vi "QueryNTPparse.vi"(0 "IP Address of NIST Server":string="132.163.4.102", 1 "error in (no error)":errorcluster) -> (2 "NTP Time":u64, 3 "time stamp UTC":timestamp, 4 "error out":errorcluster)   [LabVIEW 2012]
panel:
  out "time stamp NTP":timestamp
  out "time stamp":timestamp
  out "raw data":string
  # "This is a first draft to query an NTP server (proof of concept).\nhttp://forums.ni.com/ni/board/message?board.id=170&message.id=458949&jump=true"
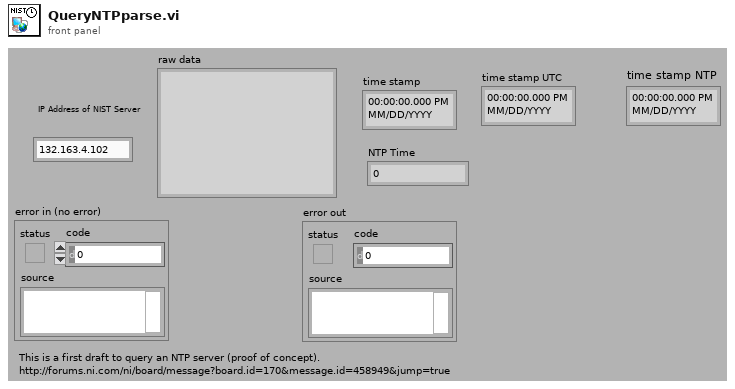
[diagram p1: front panel]
types:
  T1 = cluster{"LI|VM|Mode":u8, "Stratum":u8, "Poll":u8, "Precision":u8, "Root Delay":u32, "Root Dispersion":u32, "Reference Identifier":u32, "Reference Timestamp":fxp<+,64,32>, "Originate Timestamp":fxp<+,64,32>, "Receive Timestamp":fxp<+,64,32>, "Transmit Timestamp":fxp<+,64,32>, "Key Identifier":u32, "Message Digest-1":u64, "Message Digest-2":u64}
  T2 = typedef "LVDateTimeRec.ctl" = cluster{"fractional second":dbl, "second":i32, "minute":i32, "hour":i32, "day of month":i32, "month":i32, "year":i32, "day of week":i32, "day of year":i32, "DST":i32}
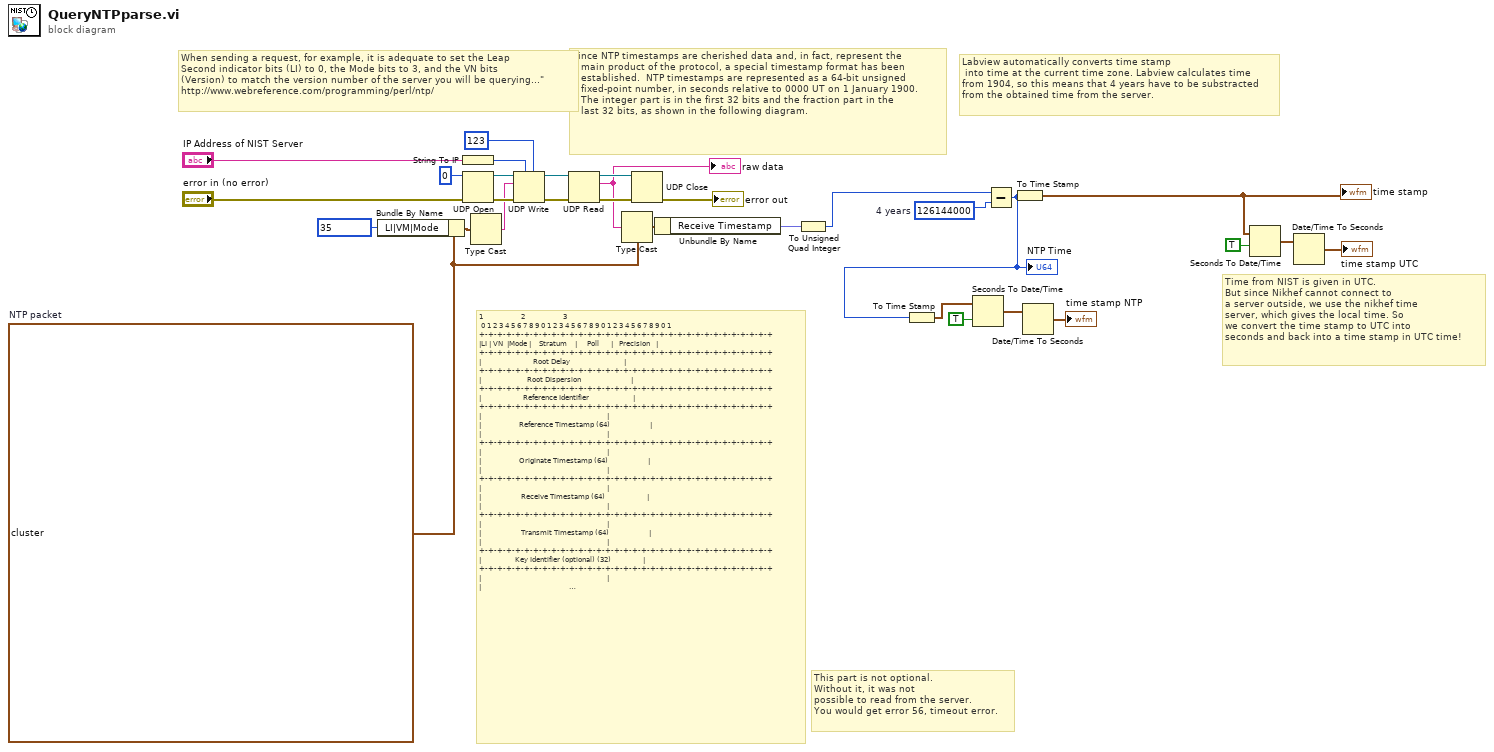
[diagram p0: block diagram]
diagram:
  w11 = T1 {"LI|VM|Mode"=0, "Stratum"=0, "Poll"=0, "Precision"=0, "Root Delay"=0, "Root Dispersion"=0, "Reference Identifier"=0, "Reference Timestamp"=0.0, "Originate Timestamp"=0.0, "Receive Timestamp"=0.0, "Transmit Timestamp"=0.0, "Key Identifier"=0, "Message Digest-1"=0, "Message Digest-2"=0}  # NTP packet
  w12 = u64 126144000  # 4 years
  # "This part is not optional.\nWithout it, it was not \npossible to read from the server.\nYou would get error 56, timeout error."
  # "Labview automatically converts time stamp\n into time at the current time zone. Labview calculates time\nfrom 1904, so this means that 4 years have to be substracted\nfrom the obtained time from the server."
  # "Time from NIST is given in UTC.\nBut since Nikhef cannot connect to\na server outside, we use the nikhef time \nserver, which gives the local time. So\nwe convert the time stamp to UTC into\nseconds and back into a time stamp in UTC time!"
  # "Since NTP timestamps are cherished data and, in fact, represent the\n   main product of the protocol, a special timestamp format has been\n   established.  NTP timestamps are represented as a 64-bit unsigned\n   fixed-point number, in seconds relative to 0000 UT on 1 January 1900.\n   The integer part is in the first 32 bits and the fraction part in the\n   last 32 bits, as shown in the following diagram."
  # "When sending a request, for example, it is adequate to set the Leap\nSecond indicator bits (LI) to 0, the Mode bits to 3, and the VN bits\n(Version) to match the version number of the server you will be querying...\"\nhttp://www.webreference.com/programming/perl/ntp/"
  # "1                   2                   3\n 0 1 2 3 4 5 6 7 8 9 0 1 2 3 4 5 6 7 8 9 0 1 2 3 4 5 6 7 8 9 0 1\n+-+-+-+-+-+-+-+-+-+-+-+-+-+-+-+-+-+-+-+-+-+-+-+-+-+-+-+-+-+-+-+-+\n|LI | VN  |Mode |    Stratum    |     Poll      |   Precision   |\n+-+-+-+-+-+-+-+-+-+-+-+-+-+-+-+-+-+-+-+-+-+-+-+-+-+-+-+-+-+-+-+-+\n|                          Root Delay                           |\n+-+-+-+-+-+-+-+-+-+-+-+-+-+-+-+-+-+-+-+-+-+-+-+-+-+-+-+-+-+-+-+-+\n|                       Root Dispersion                         |\n+-+-+-+-+-+-+-+-+-+-+-+-+-+-+-+-+-+-+-+-+-+-+-+-+-+-+-+-+-+-+-+-+\n|                     Reference Identifier                      |\n+-+-+-+-+-+-+-+-+-+-+-+-+-+-+-+-+-+-+-+-+-+-+-+-+-+-+-+-+-+-+-+-+\n|                                                               |\n|                   Reference Timestamp (64)                    |\n|                                                               |\n+-+-+-+-+-+-+-+-+-+-+-+-+-+-+-+-+-+-+-+-+-+-+-+-+-+-+-+-+-+-+-+-+\n|                                                               |\n|                   Originate Timestamp (64)                    |\n|                                                               |\n+-+-+-+-+-+-+-+-+-+-+-+-+-+-+-+-+-+-+-+-+-+-+-+-+-+-+-+-+-+-+-+-+\n|                                                               |\n|                    Receive Timestamp (64)                     |\n|                                                               |\n+-+-+-+-+-+-+-+-+-+-+-+-+-+-+-+-+-+-+-+-+-+-+-+-+-+-+-+-+-+-+-+-+\n|                                                               |\n|                    Transmit Timestamp (64)                    |\n|                                                               |\n+-+-+-+-+-+-+-+-+-+-+-+-+-+-+-+-+-+-+-+-+-+-+-+-+-+-+-+-+-+-+-+-+\n|                 Key Identifier (optional) (32)                |\n+-+-+-+-+-+-+-+-+-+-+-+-+-+-+-+-+-+-+-+-+-+-+-+-+-+-+-+-+-+-+-+-+\n|                                                               |\n|                                                               |\n|                 Message Digest (optional) (128)               |\n|                                                               |\n|                                                               |\n+-+-+-+-+-+-+-+-+-+-+-+-+-+-+-+-+-+-+-+-+-+-+-+-+-+-+-+-+-+-+-+-+"
  n1 = Bundle By Name(cluster=w11, "LI|VM|Mode"=u8 35) -> (w13:T1)
  n2 = String To IP(1:"IP Address of NIST Server") -> (0:w25:u32)
  n3 = UDP Open(8:"error in (no error)", 11:u16 0 ("port")) -> (port=w27:refnum<k16>, 0:w24:errorcluster)  [unwired: 3 in, 1 out]
  n4 = Type Cast(x=w13) -> (*(type *) &x=w20:string)  [unwired: 1 in]
  n5 = UDP Write(address=w25, port or service name=u16 123, connection ID=w27, data in=w20, 8:w24) -> (error out=w23:errorcluster, 3:w28:refnum<k16>)  [unwired: 1 in]
  n6 = UDP Read(connection ID=w28, 8:w23) -> (data out=w17:string, error out=w30:errorcluster, 3:w29:refnum<k16>)  [unwired: 2 in, 2 out]
  "raw data" <- w17
  n7 = Type Cast(type=w11, x=w17) -> (*(type *) &x=w16:T1)
  n8 = UDP Close(connection ID=w29, 8:w30) -> (error out=→"error out":errorcluster)  [unwired: 1 out]
  n9 = Unbundle By Name(w16) -> ("Receive Timestamp"=w15:fxp<+,64,32>)
  n10 = To Unsigned Quad Integer(1:w15) -> (0:w2:u64)
  n11 = Subtract(x=w2, y=w12) -> (x-y=w1:u64)
  "NTP Time" <- w1
  n12 = To Time Stamp(1:w1) -> (0:w5:timestamp)
  n13 = Seconds To Date/Time(time stamp (now)=w5, to UTC (F)=TRUE) -> (date time rec=w4:T2)
  n14 = To Time Stamp(1:w1) -> (0:w8:timestamp)
  "time stamp" <- w8
  n15 = Date/Time To Seconds(2:w4) -> (0:→"time stamp NTP":timestamp)  [unwired: 1 in]
  n16 = Seconds To Date/Time(time stamp (now)=w8, to UTC (F)=TRUE) -> (date time rec=w10:T2)
  n17 = Date/Time To Seconds(2:w10) -> (0:→"time stamp UTC":timestamp)  [unwired: 1 in]
